vi "GetWL.vi"(3 "error in (no error)":errorcluster, 4 "Integration Time":i32, 5 "Type":T1, 6 "USB4000 Params In":T2) -> (0 "error out":errorcluster, 1 "Saturated?":bool, 2 "USB4000 Params Out":T2)   [LabVIEW 2012]
uses:
  Controls/USB4000_Data.ctl
  Classes/Controls/SpectrometerOphirSelector.ctl
panel:
  out "EL spectrum":dbl[](array[numeric])
  out "Wavelength":dbl[](array[numeric]) format="%.2f"
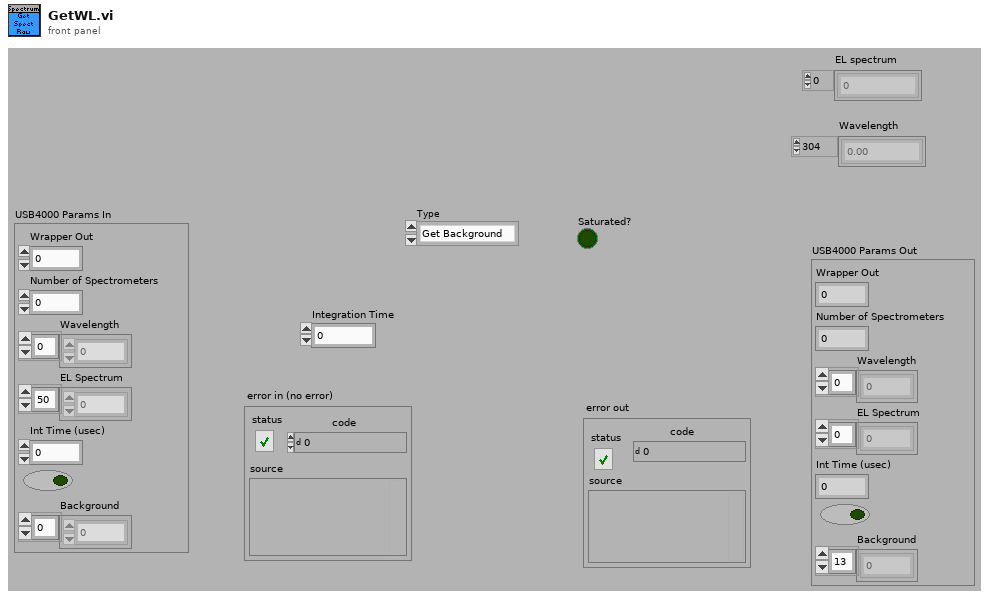
[diagram p1: front panel]
types:
  T1 = typedef "SpectrometerOphirSelector.ctl" = enum16{"Get Background", "Measure", "Measure50", "Raw"}
  T2 = typedef "USB4000_Data.ctl" = cluster{"Wrapper Out":u32, "Number of Spectrometers":i32, "Wavelength":dbl[], "EL Spectrum":dbl[], "Int Time (usec)":i32, bool, "Background":dbl[]}
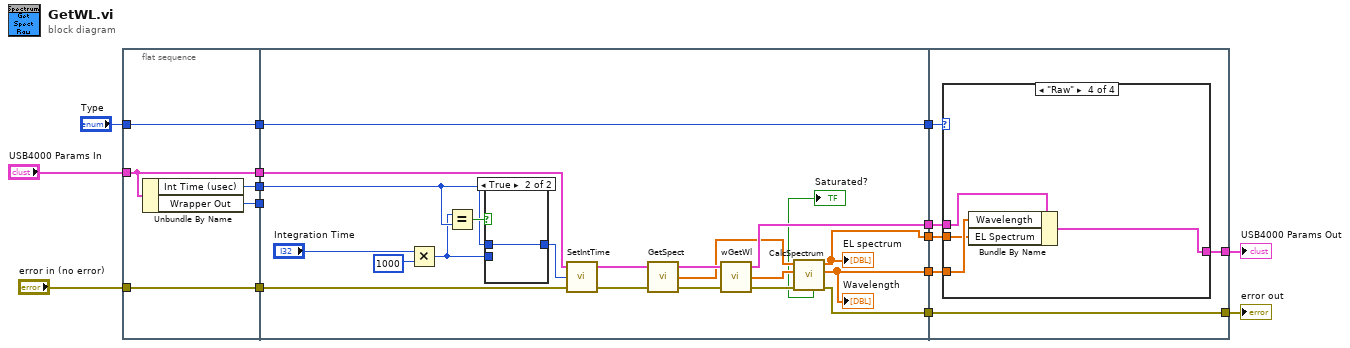
[diagram p0: block diagram]
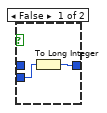
[diagram p2: hidden frame]
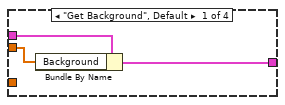
[diagram p3: hidden frame]
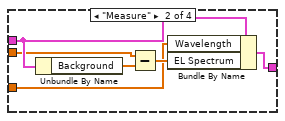
[diagram p4: hidden frame]
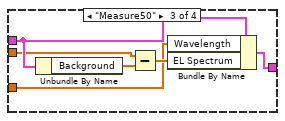
[diagram p5: hidden frame]
diagram:
  n1 = flat-sequence {
    tunnel: "error in (no error)" -> [w17]
    tunnel: [w19] -> w12
    tunnel: [w20] -> w11
    tunnel: [w17] -> w10
    tunnel: "USB4000 Params In" -> [w18]
    tunnel: [w18] -> w7
    tunnel: [w16] -> w4
    tunnel: "Type" -> [w16]
    tunnel: [w22] -> w15
    tunnel: [w28] -> w8
    tunnel: [w41] -> w5
    tunnel: w4 -> [w41]
    tunnel: w7 -> [w35]
    tunnel: w10 -> [w34]
    tunnel: w11 -> [w37]
    tunnel: w12 -> [_]
    tunnel: [w26] -> w2
    tunnel: [w23] -> w1
    tunnel: w15 -> [w50]
    tunnel: w8 -> [w46]
    tunnel: [w48] -> w6
    tunnel: [w47] -> w13
    tunnel: w5 -> [w45]
    tunnel: w2 -> [w48]
    tunnel: w1 -> [w49]
    frame #0 {
      n2 = Unbundle By Name(w18) -> ("Int Time (usec)"=w20:i32, "Wrapper Out"=w19:u32)
    }
    frame #1 {
      n3 = Multiply(x="Integration Time", y=1000) -> (x*y=w36:i32)
      n4 = Equal?(x=w36, y=w37) -> (x = y?=w38:bool)
      n5 = case shown="True" w38 {
        tunnel: [w42 w44] -> w33
        tunnel: w37 -> [_ w44]
        tunnel: w36 -> [w43 _]
        frame False {
          n6 = To Long Integer(number=w43) -> (32bit integer=w42:i32)
        }
        frame True {
        }
      }
      n7 = call "SetIntTime.vi"("error in"=w34, "Integration Time"=w33, "SpectRef In"=w35) -> ("error out"=w31:errorcluster, "SpectRef Out"=w32:T2)  [unwired: 1 in]
      n8 = call "GetSpect.vi"("error in (no error)"=w31, "SpectRef In"=w32) -> ("error out"=w29:errorcluster, "Spectrum Values"=w24:dbl[], "SpectRef Out"=w30:T2)  [unwired: 1 in]
      n9 = call "wGetWl.vi"("error in (no error)"=w29, "SpectRef In"=w30) -> ("error out"=w27:errorcluster, "WL Values"=w25:dbl[], "SpectRef Out"=w28:T2)  [unwired: 1 in]
      n10 = call "CalcSpectrum.vi"("error in (no error)"=w27, "Wavelength"=w25, "Spectrum"=w24) -> ("error out"=w26:errorcluster, "WavelengthSplit"=w22:dbl[], "SpectrumSplit"=w23:dbl[], "Saturated?"=→"Saturated?":bool)  [unwired: 3 in, 2 out]
      "EL spectrum" <- w23
      "Wavelength" <- w22
    }
    frame #2 {
      n11 = case shown="\"Raw\"" w45 {
        tunnel: w46 -> [w53 w59 w65 w68]
        tunnel: w50 -> [_ w54 w60 w67]
        tunnel: w49 -> [w52 w57 w63 w66]
        tunnel: [w51 w55 w61 w69] -> w47
        frame "Get Background", Default {
          n12 = Bundle By Name(cluster=w53, "Background"=w52) -> (w51:T2)
        }
        frame "Measure" {
          n13 = Unbundle By Name(w59) -> ("Background"=w58:dbl[])
          n14 = Subtract(x=w57, y=w58) -> (x-y=w56:dbl[])
          n15 = Bundle By Name(cluster=w59, "Wavelength"=w54, "EL Spectrum"=w56) -> (w55:T2)
        }
        frame "Measure50" {
          n16 = Unbundle By Name(w65) -> ("Background"=w64:dbl[])
          n17 = Subtract(x=w63, y=w64) -> (x-y=w62:dbl[])
          n18 = Bundle By Name(cluster=w65, "Wavelength"=w60, "EL Spectrum"=w62) -> (w61:T2)
        }
        frame "Raw" {
          n19 = Bundle By Name(cluster=w68, "Wavelength"=w67, "EL Spectrum"=w66) -> (w69:T2)
        }
      }
    }
  }
  "USB4000 Params Out" <- w13
  "error out" <- w6
